vi "Array.vi"(11 "data":dynamicdata(waveform)) -> (3 "Array":dynamicdata[][](array[waveform]))   [LabVIEW 2011]
panel:
  in  "Numeric":i32
  out "Multicolumn Listbox":i32(listbox)
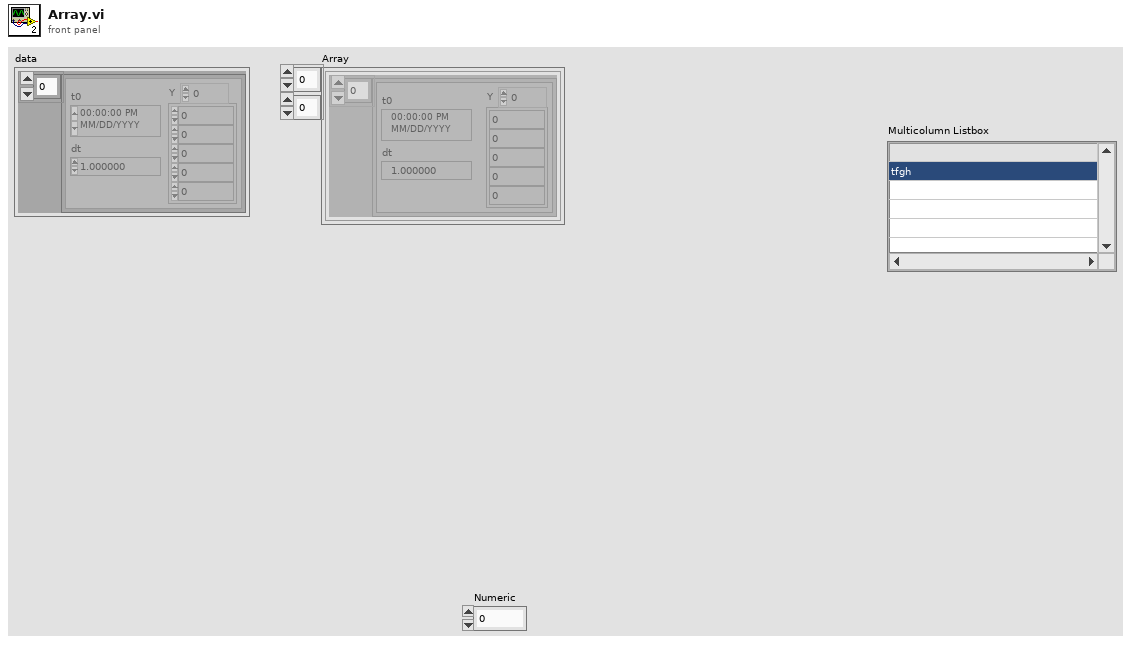
[diagram p1: front panel]
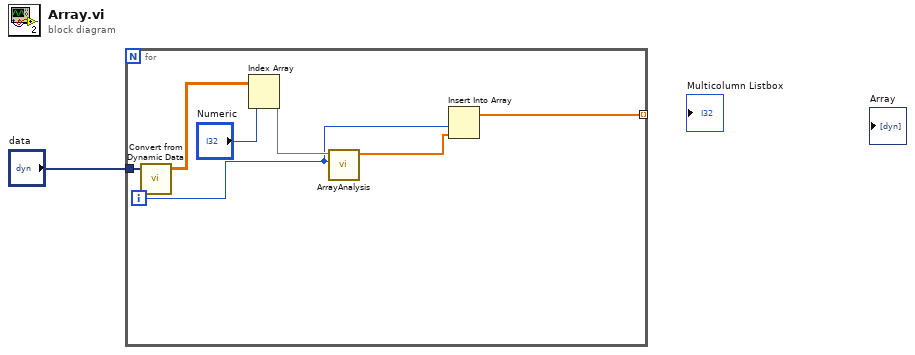
[diagram p0: block diagram]
diagram:
  n1 = for {
    tunnel: "data" -> [w8]
    tunnel: [w2] -> _ mode=indexing
    i -> [w4]
    n2 = call "Convert from Dynamic Data"("Dynamic Data Type"=w8) -> ("Array"=w6:dbl[][])  [unwired: 3 in]
    n3 = Index Array(array=w6, index (row)="Numeric") -> (element=w5:dbl[])  [unwired: 1 in]
    n4 = call "ArrayAnalysis.vi"("Numeric"=w4, "Array in"=w5) -> ("Array out"=w3:dbl[])  [unwired: 9 in]
    n5 = Insert Into Array(index=w4, new element=w3) -> (w2:dbl[])  [unwired: 1 in]
  }
